vi "test Block Upload C5-E.vi"(11 "Test Case In":refnum<class "Tests SDO Manager.lvclass">) -> (0 "error out":errorcluster, 3 "Test Case Out":refnum<class "Tests SDO Manager.lvclass">)   [LabVIEW 2020, in "Tests SDO Manager.lvclass"]
uses:
  Tests SDO Manager.lvclass
  source/Logging/Logger/Logger.lvclass
  HAL/Source/Communicator/Communicator.lvclass
  <vilib>/ActorFramework/Stop Msg/Stop Msg.lvclass
  HAL/HAL-Devices/source/PCAN USB Dongle/PCAN Basic 4/Configure Strategies/Read-Write CAN Frame Strategy/PCAN Basic4 Read-Write CAN CC Frame Strategy.lvclass
  HAL/Source/Interfaces/IMessage/IMessage.lvclass
  Tests SDO Manager.lvclass/Tests SDO Manager.ctl
  D:/git/HAL/HAL-Devices/source/PCAN USB Dongle/PCAN Basic 4/Configure Strategies/Base Configure Strategy/PCAN Basic4 Base Configure Strategy.lvclass
  D:/git/HAL/Source/Interfaces/IApplyConfiguration/IApplyConfiguration.lvclass
  D:/git/HAL/Source/Interfaces/IClose/IClose.lvclass
  D:/git/HAL/Source/Interfaces/IInitialize/IInitialize.lvclass
  D:/git/HAL/Source/Interfaces/ICommunicate/ICommunicate.lvclass
  D:/git/HAL/Source/Interfaces/IRunnable/IRunnable.lvclass
  D:/git/HAL/Source/Interfaces/IValidate Configuration/IValidate Configuration.lvclass
  D:/git/HAL/HAL-Devices/source/PCAN USB Dongle/PCAN Basic 4/Configure Strategies/Read-Write CAN Frame Strategy/PCAN Basic4 Read-Write CAN CC Frame Strategy.lvclass
  D:/git/HAL/Source/Interfaces/IInstrument/IInstrument.lvclass
  D:/git/HAL/Source/Communicator/Communicator.lvclass
  D:/git/HAL/Source/Interfaces/IConfigurable/IConfigurable.lvclass
  C:/Program Files/National Instruments/LabVIEW 2026/vi.lib/ActorFramework/Actor/Actor.lvclass
  D:/git/CANopen-LabVIEW/source/Logging/Logger/Logger.lvclass
  4993e8ee-a06a-463a-9684-69129f64d5ce.vi
  source/SDO/SDO Manager/SDO Manager/SDO Manager.lvclass
  source/Logging/Log Level.vi
  source/Logging/CANopen Logging.lvlib
  <vilib>/ActorFramework/Actor/Actor.lvclass
  source/SDO/SDO Manager/SDO Transfer/SDO abort code.ctl
  source/SDO/SDO Manager/SDO Transfer/SDO Transfer.lvclass
  source/Typedefs/SDO Result.ctl
panel:
  out "size(s)":i32
  out "Data.Data":u8[](array[numeric])
  out "SDO Result":T1={"Success"=FALSE, "SDO abort code"={"Null"=TRUE, "Value"=84082688}, "Data"={"Null"=TRUE, "Data"=[]}} {"SDO abort code"."Value" items=["Toggle bit not allowed"=84082688, "SDO protocol timed out"=84148224, "Client/server command specifier not valid or unknown"=84148225, "Invalid block size (block mode only)"=84148226, "Invalid sequence number (block mode only)"=84148227, "CRC error (block mode only)"=84148228, "Out of memory"=84148229, "Attempt to read a write only object"=100728833, "Attempt to write a read only object"=100728834, "Object does not exist in the object dictionary"=100794368, "Object cannot be mapped to the PDO"=100925505, "The number and length of the objects to be mapped would exceed PDO length"=100925506, "General parameter incompatibility reason"=100925507, "General internal incompatibility in the device"=100925511, "Access failed due to an hardware error"=101056512, "Data type does not match, length of service parameter does not match"=101122064, "Data type does not match, length of service parameter too high"=101122066, "Data type does not match, length of service parameter too low"=101122067, "Sub-index does not exist"=101253137, "Invalid value for parameter (download only)"=101253168, "Value of parameter written too high (download only)"=101253169, "Value of parameter written too low (download only)"=101253170, "Maximum value is less than minimum value"=101253174, "Resource not available: SDO connection"=101318691, "General error"=134217728, "Data cannot be transferred or stored to the application"=134217760, "Data cannot be transferred or stored to the application because of local control"=134217761, "Data cannot be transferred or stored to the application because of the present device stable"=134217762, "Object dictionary dynamic generation fails or no object dictionary is present (e.g. object dictionary is generated from file and generation fails because of an file error)"=134217763, "No data available"=134217764]; "Data"."Data" format="%02x"}
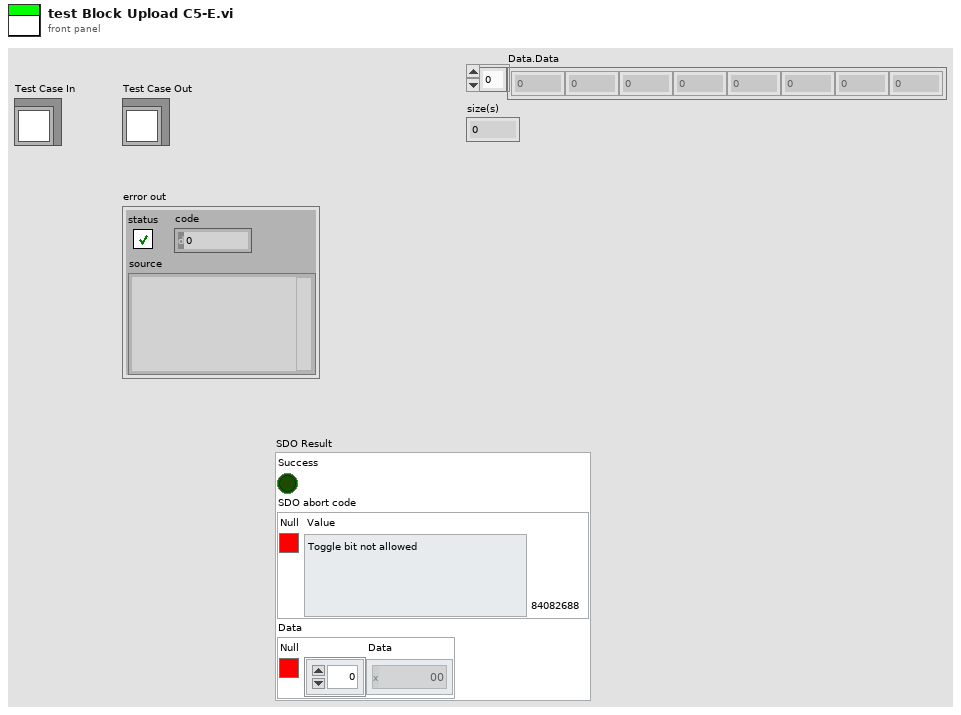
[diagram p1: front panel]
types:
  T1 = typedef "CANopen.lvlib/SDO Manager.lvlib/SDO Transfer.lvclass/SDO Result.ctl" = cluster{"Success":bool, "SDO abort code":cluster{"Null":bool, "Value":T2}, "Data":cluster{"Null":bool, "Data":u8[]}}
  T2 = typedef "CANopen.lvlib/SDO Manager.lvlib/SDO Transfer.lvclass/SDO abort code.ctl" = u32
  T3 = cluster{"Node-ID":u8, "Multiplexer":cluster{"Index":u16, "Sub-Index":u8}, "Data":u8[]}
  T4 = enum16{"Error", "Warn", "Info", "Debug", "Trace"}
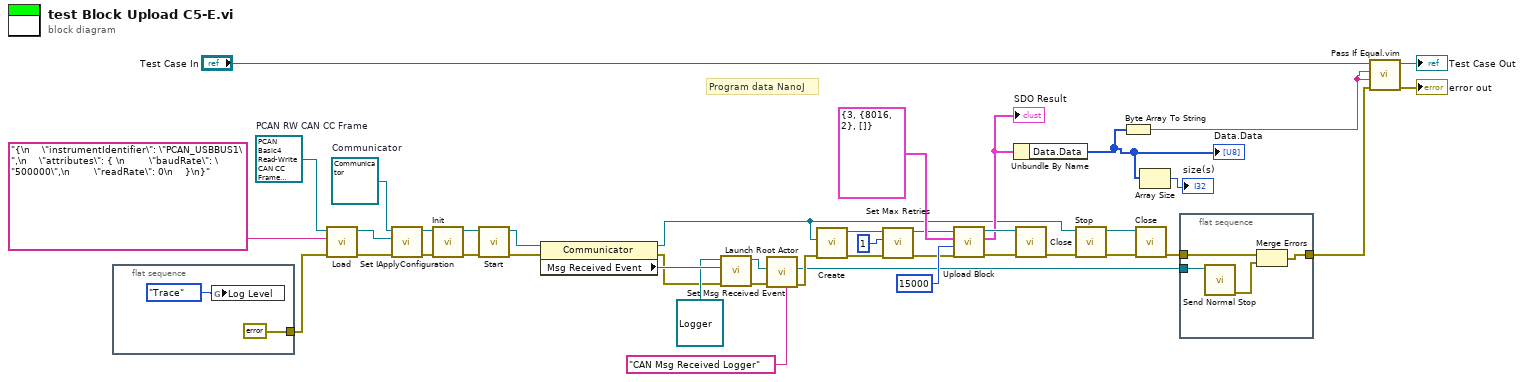
[diagram p0: block diagram]
diagram:
  w9 = refnum<class "Communicator.lvclass"> refnum  # Communicator
  w16 = refnum<class "PCAN Basic4 Read-Write CAN CC Frame Strategy.lvclass"> refnum  # PCAN RW CAN CC Frame
  # "Program data NanoJ"
  n1 = flat-sequence {
    tunnel: [errorcluster {"status"=FALSE, "code"=0, "source"=""} ("error constant")] -> w14
    frame #0 {
      n2 = global write "Log Level.vi" "Log Level"(T4."Trace" ("Log Level")) -> ()
    }
  }
  n3 = call-dynamic "Load.vi"("error in"=w14, "Source"="{\n    \"instrumentIdentifier\": \"PCAN_USBBUS1\",\n    \"attributes\": { \n        \"baudRate\": \"500000\",\n        \"readRate\": 0\n    }\n}", "PCAN Basic Base Configure Strategy in"=w16) -> ("error out"=w12:errorcluster, "PCAN Basic Base Configure Strategy out"=w13:refnum<class "PCAN Basic4 Read-Write CAN CC Frame Strategy.lvclass">)  [unwired: 7 in]
  n4 = call-dynamic "Set IApplyConfiguration.vi"("Error In"=w12, "IÁpplyConfiguration"=w13, "Communicator in"=w9) -> ("Error Out"=w11:errorcluster, "Communicator out"=w10:refnum<class "Communicator.lvclass">)  [unwired: 7 in]
  n5 = call-dynamic "Init.vi"("Error In"=w11, "Communicator in"=w10) -> ("Error Out"=w8:errorcluster, "Communicator out"=w7:refnum<class "Communicator.lvclass">)  [unwired: 8 in]
  n6 = call-dynamic "Start.vi"("Error In"=w8, "Communicator in"=w7) -> ("Error Out"=w6:errorcluster, "Communicator out"=w5:refnum<class "Communicator.lvclass">)  [unwired: 8 in]
  n7 = property class="Communicator"(reference=w5, error in=w6) -> (reference out=w1:refnum<class "Communicator.lvclass">, error out=w4:errorcluster, "Msg Received Event"=w31:refnum<user-event>)
  n8 = call "Set Msg Received Event.vi"("error in"=w4, "Msg Received Event"=w31, "Logger in"=refnum<class "Logger.lvclass"> refnum) -> ("error out"=w33:errorcluster, "Logger out"=w32:refnum<class "Logger.lvclass">)  [unwired: 7 in]
  n9 = call <vilib>:"Launch Root Actor.vi"("Debug Alias"="CAN Msg Received Logger", "error in (no error)"=w33, "Actor"=w32) -> ("error out"=w30:errorcluster, "Actor's Enqueuer"=w27:refnum<class "Message Enqueuer.lvclass">)  [unwired: 7 in]
  n10 = call "Create.vi"("Error In"=w30, "ICommunicate"=w1) -> ("Error Out"=w25:errorcluster, "SDO Manager"=w24:refnum<class "SDO Manager.lvclass">)  [unwired: 8 in]
  n11 = call "Set Max Retries.vi"("error in"=w25, "Max Retries"=u8 1, "SDO Manager in"=w24) -> ("error out"=w22:errorcluster, "SDO Manager out"=w23:refnum<class "SDO Manager.lvclass">)  [unwired: 7 in]
  n12 = call "Upload Block.vi"("error in"=w22, "Timeout"=15000, "Parameters"=T3 {"Node-ID"=3, "Multiplexer"={"Index"=8016, "Sub-Index"=2}, "Data"=[]}, "SDO Manager in"=w23) -> ("error out"=w37:errorcluster, "SDO Result"=w34:T1, "SDO Manager out"=w36:refnum<class "SDO Manager.lvclass">)  [unwired: 5 in]
  "SDO Result" <- w34
  n13 = Unbundle By Name(w34) -> ("Data.Data"=w19:u8[])
  "Data.Data" <- w19
  n14 = call "Close.vi"("Error In"=w37, "SDO Manager"=w36) -> ("Error Out"=w39:errorcluster)  [unwired: 8 in, 1 out]
  n15 = call-dynamic "Stop.vi"("Error In"=w39, "Communicator in"=w1) -> ("Error Out"=w3:errorcluster, "Communicator out"=w2:refnum<class "Communicator.lvclass">)  [unwired: 8 in]
  n16 = Byte Array To String(unsigned byte array=w19) -> (string=w20:string)
  n17 = call-dynamic "Close.vi"("Error In"=w3, "Communicator in"=w2) -> ("Error Out"=w28:errorcluster)  [unwired: 8 in, 1 out]
  n18 = Array Size(array=w19) -> (size(s)=→"size(s)":i32)
  n19 = flat-sequence {
    tunnel: w28 -> [w45]
    tunnel: w27 -> [w48]
    tunnel: [w46] -> w26
    frame #0 {
      n20 = call <vilib>:"Send Normal Stop.vi"("Message Enqueuer"=w48) -> ("error out"=w47:errorcluster)  [unwired: 10 in]
      n21 = Merge Errors(w45, w47) -> (w46:errorcluster)
    }
  }
  n22 = call "Pass If Equal.vim"("error in (no error)"=w26, "Actual"=w20, "Expected"=w20, "LUnit Test Case In"="Test Case In") -> ("error out"=→"error out":errorcluster, "LUnit Test Case Out"=→"Test Case Out":refnum<class "Tests SDO Manager.lvclass">)  [unwired: 6 in]
